vi "Get Breakpoints Lines Numbers.vi"(10 "wires with breakpoints":string[](array[string]), 11 "transcripted code":string) -> (3 "breakpoints lines numbers":i32[](array[numeric]))   [LabVIEW 2014]
doc: "Returns array of numbers of lines in source code where should be placed breakpoints. This VI takes as input labels of wires and is looking where in source code are located (but no declaration of wires, but their usage like assignement) and return first occurence of wire usage.\nThis is used for debugging MCU by external tools to know where to place breakpoints in source code."
uses:
  <vilib>/regexp/Match Regular Expression.xnode
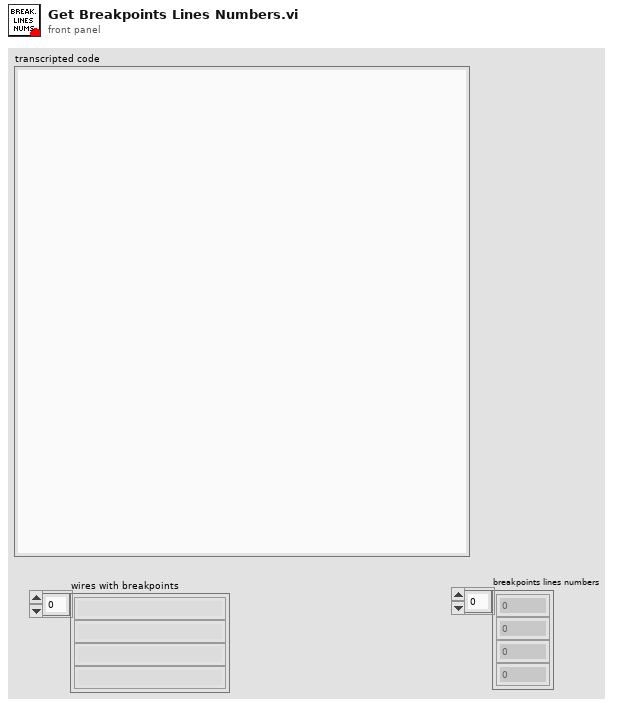
[diagram p1: front panel]
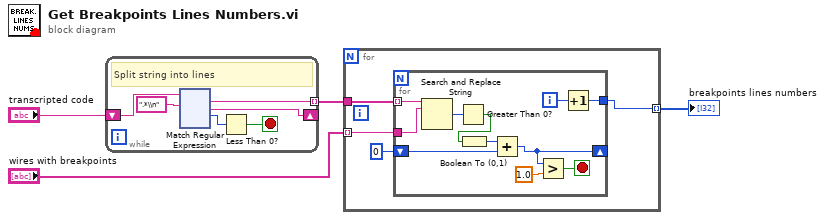
[diagram p0: block diagram]
diagram:
  n1 = while {
    tunnel: [w6] -> w3 mode=indexing
    shift-right: [w5] -> _
    shift-left: "transcripted code" -> [w10]
    stop <- w7 stop-if-true
    # "Split string into lines"
    n2 = xnode "Match Regular Expression"("input string"=w10, "regular expression"=".*\\n") -> ("whole match"=w6:string, "after match"=w5:string, "offset past match"=w8:i32)  [unwired: 4 in, 2 out]
    n3 = Less Than 0?(x=w8) -> (x < 0?=w7:bool)
  }
  n4 = for {
    tunnel: w3 -> [w127]
    tunnel: "wires with breakpoints" -> [w128] mode=indexing
    tunnel: [w125] -> w1 mode=indexing
    n5 = for {
      tunnel: w128 -> [w138]
      tunnel: w127 -> [w139] mode=indexing
      shift-right: [w131] -> _
      shift-left: 0 -> [w134]
      tunnel: [w129] -> w125
      i -> [w130]
      stop <- w133 stop-if-true
      n6 = Search and Replace String(input string=w139, search string=w138) -> (number of replacements=w137:i32)  [unwired: 6 in, 3 out]
      n7 = Greater Than 0?(x=w137) -> (x > 0?=w136:bool)
      n8 = Boolean To (0,1)(Boolean=w136) -> (0, 1=w135:i16)
      n9 = Add(x=w135, y=w134) -> (x+y=w131:i32)
      n10 = Greater?(x=w131, y=1.0) -> (0:w133:bool)
      n11 = Increment(x=w130) -> (x+1=w129:i32)
    }
  }
  "breakpoints lines numbers" <- w1
